vi "batch processor.vi"() -> ()   [LabVIEW 2012]
uses:
  <vilib>/Utility/miscctls.llb/LVPointTypeDef.ctl
  Private/File_location.ctl
  Public API/Post_Dust_Event.ctl
  Private/Estimate_source.ctl
  <vilib>/Utility/error.llb/DialogType.ctl
  Public API/Signal.ctl
  Private/Role ID.ctl
  Private/Hardware ID.ctl
panel:
  in  "stop 2":bool
  in  "Tab Control":enum32{"Controls", "Processing"}(tab)
  in  "Update old Errored entries?":bool
  in  "Clear IDL Errors 2":bool
  in  "Clear IDL Errors":bool
  out "Warning:":string
  out "Move Errors":errorcluster
  out "IDL Errors":errorcluster
  out "Test":bool caption="Test Database in use:"
  out "Test 2":bool=TRUE caption="Production Database in use:"
  out "Events being processed:":i32
  out "Processing Frequency (Hz):":dbl
  out "Database Update Progress:":u8(slide) scale=0.0..100.0
  out "IDL Code Executing":bool=TRUE
  out "Estimated IDL Progress:":u8(slide) scale=0.0..100.0
  in  "Update old database entries?":bool
  in  "Upper Timestamp\nFor Old Data":timestamp
  in  "Lower Timestamp\nFor Old Data":timestamp
  out "Running Old Data:":bool
  out "standard error":string
  out "standard output":string
  out "Passed":i32
  out "Quality":ext format="%.2f"
  out "Charge":ext
  out "Velocity":ext
  out "Source":i32
  out "Time taken by IDL per shot: (s)":dbl
  out "Shot being processed:":string
  out "Remaining Shots:":string
  out "Output to IDL command line:":string
  in  "stop":bool
  out "Radius":dbl
  out "Mass":ext
  out "Dust Event ID":i64
  out "High Voltage":sgl
  # "CCLDAS Database Update System V1.0"
  # "Error Status:"
  # "Beamline length change: 1:00:00.000 PM\n                                                       3/5/2014"
  # "ODBC Connection Status:"
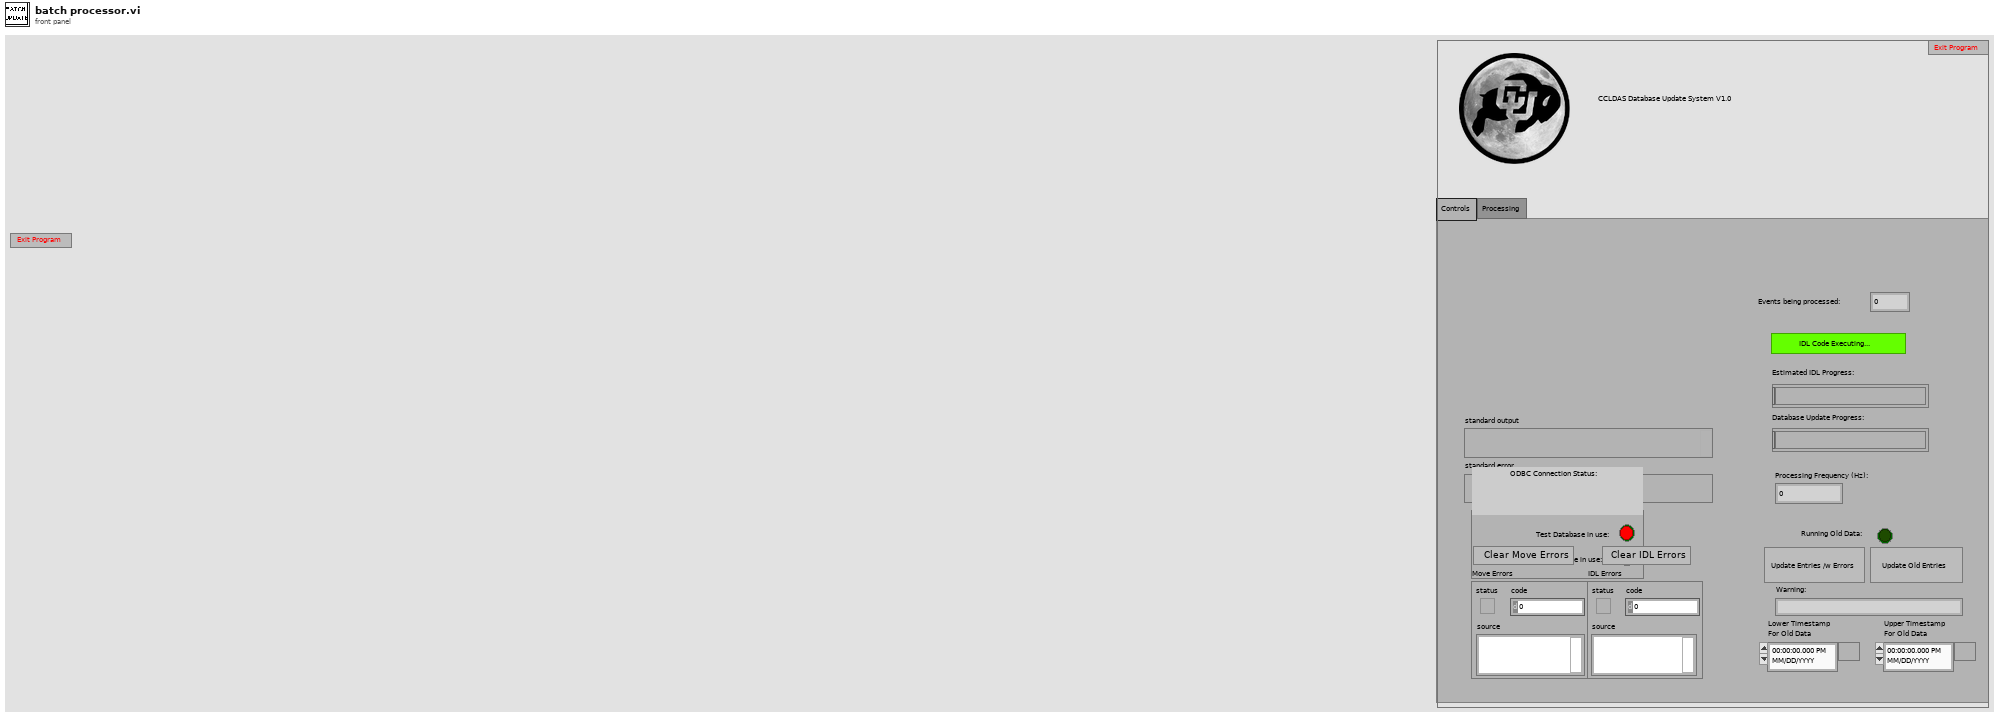
[diagram p1: front panel]
types:
  T1 = typedef "LVPointTypeDef.ctl" = cluster{"Horizontal":i16, "Vertical":i16}
  T2 = enum16{"open", "replace", "create", "open or create", "replace or create", "replace or create with confirmation"}
  T3 = typedef "Post_Dust_Event.ctl" = cluster{"Dust Event ID":i64, "Integer Timestamp":i64, "Velocity":sgl, "Mass":sgl, "Charge":sgl, "Radius":sgl, "Passed_3rd_Detector":i8, "Experiment Settings":dbl, "Pelletron ID":i32, "Estimate Source":T4, "Estimate Quality":sgl, "File Location":T5, "id_dust_info":dbl}
  T4 = typedef "Estimate_source.ctl" = i8
  T5 = typedef "File_location.ctl" = i8
  T6 = typedef "bp_cluster.ctl" = cluster{"Dust Event ID":i64, "High Voltage":sgl, "Experiment Settings  ID":i64, "File Location":T5, "Dust Density":dbl}
  T7 = enum8{"Enabled", "Disabled", "Disabled and Grayed Out"}
  T8 = typedef "Signal.ctl" = cluster{"Signal ID":i64, "Time Stamp":timestamp, "Dust Event ID":i64, "Role ID":T9, "Data":sgl[], "Signal Length":i32, "dt":sgl, "Offset":dbl, "Hardware ID":T10}
  T9 = typedef "Role ID.ctl" = enum16{"First_Detector", "Second_Detector", "Third_Detector", "LeCroy_CH1", "LeCroy_CH2", "LeCroy_CH3", "LeCroy_CH4", "PSU"}
  T10 = typedef "Hardware ID.ctl" = enum16{"Unknown", "CSA 1", "CSA 2", "CSA 3", "CSA 4", "CSA 5", "CSA 6"}
  T11 = typedef "DialogType.ctl" = u16
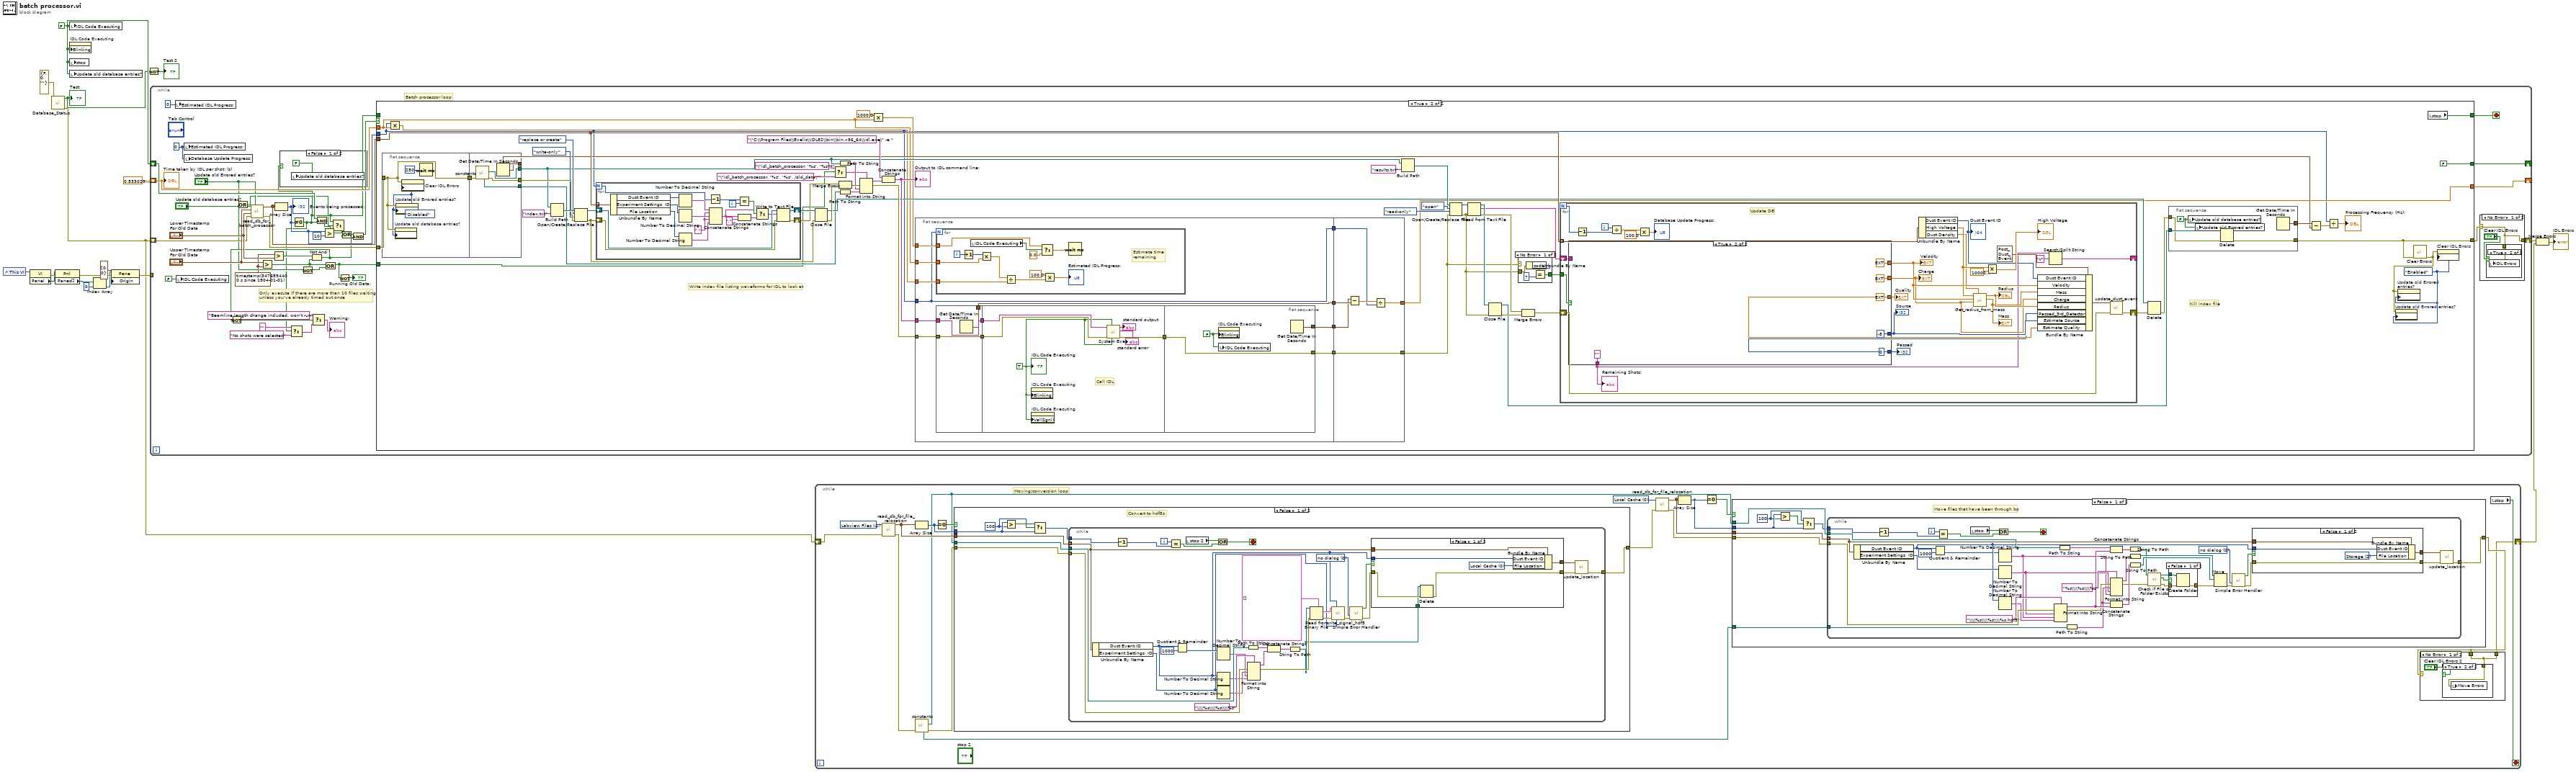
[diagram p0: block diagram]
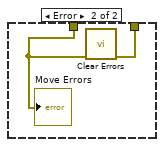
[diagram p3: hidden frame]
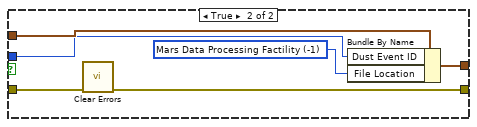
[diagram p4: hidden frame]
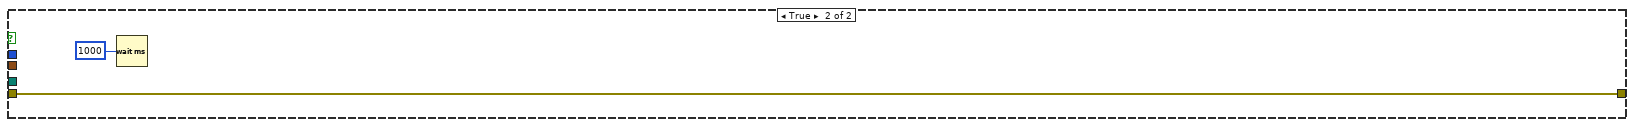
[diagram p5: hidden frame]
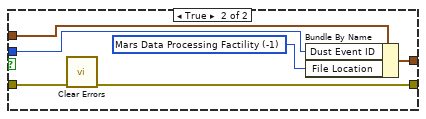
[diagram p6: hidden frame]
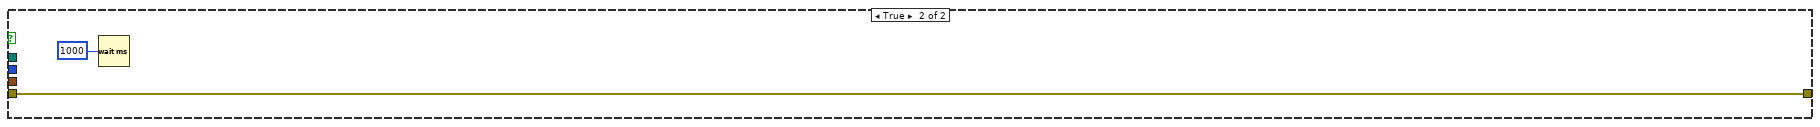
[diagram p8: hidden frame]
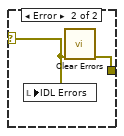
[diagram p10: hidden frame]
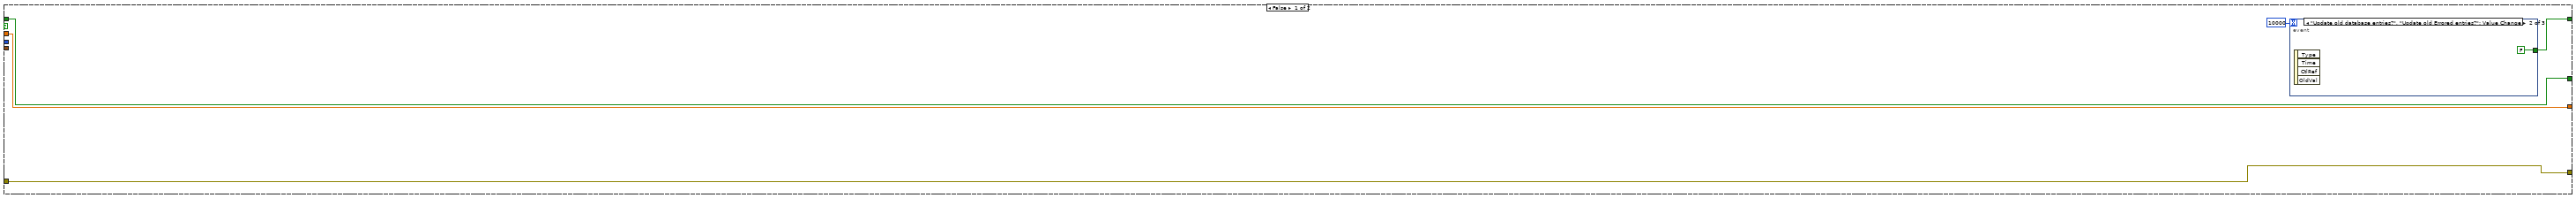
[diagram p12: hidden frame]
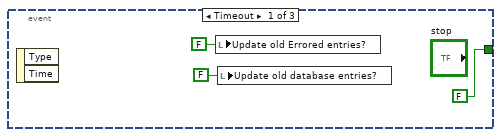
[diagram p13: hidden frame]
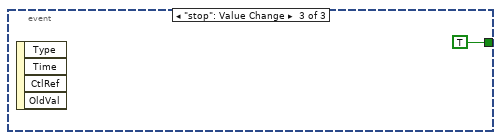
[diagram p14: hidden frame]
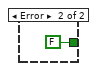
[diagram p15: hidden frame]
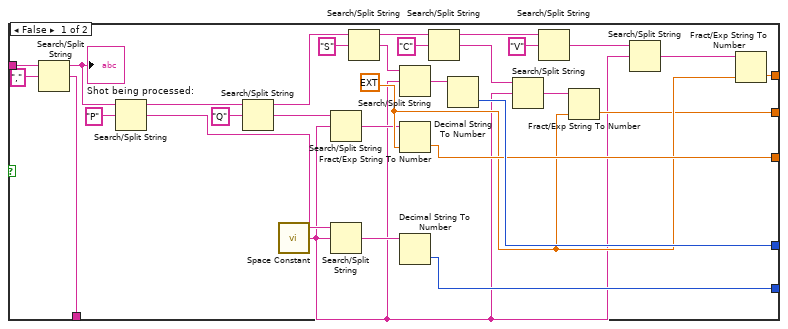
[diagram p16: hidden frame]
diagram:
  w18 = FALSE ("IDL Code Executing")
  n1 = control-ref of="This VI"() -> (w13:refnum<vi>)
  n2 = property class="VI"(reference=w13) -> (error out=w12:errorcluster, "Panel"=w11:refnum<vi>)  [unwired: 1 in, 1 out]
  n3 = call "Database_Status.vi"("error in (no error)"=errorcluster {"status"=FALSE, "code"=0, "source"=""}) -> ("error out"=w3:errorcluster, "Test Database"=w15:bool)  [unwired: 9 in]
  "Test" <- w15
  n4 = property class="Pnl"(reference=w11, error in=w12) -> (error out=w10:errorcluster, "Panes[]"=w9:refnum<vi>[])  [unwired: 1 out]
  n5 = local write "IDL Code Executing"(w18) -> ()
  n6 = property on="IDL Code Executing" class="Bool (strict)"("Blinking"=w18) -> ()  [unwired: 2 in, 2 out]
  n7 = local write "stop"(w18) -> ()
  n8 = local write "Update old database entries?"(w18) -> ()
  n9 = Index Array(array=w9, index=0) -> (element=w7:refnum<vi>)
  n10 = property class="Pane"(reference=w7, error in=w10, "Origin"=T1 {"Horizontal"=0, "Vertical"=0}) -> (error out=w5:errorcluster)  [unwired: 1 out]
  n11 = Not(x=w15) -> (.not. x?=→"Test 2":bool)
  n12 = while {
    shift-right: [w52] -> _
    shift-left: sgl 0.53303 ("y") -> [w53]
    shift-right: [w47] -> _
    shift-left: w18 -> [w48]
    tunnel: w5 -> [_]
    shift-right: [w19] -> w2
    shift-left: w3 -> [w28]
    stop <- w50 stop-if-true
    w42 = timestamp(3476894400 s since 1904-01-01) ("y")
    w54 = u8 0 ("Database Update Progress")
    # "Only execute if there are more than 10 files waiting \nunless you've already timed out once"
    # "Batch processor loop"
    n13 = local write "Estimated IDL Progress:"(u8 0 ("Estimated IDL Progress")) -> ()
    n14 = local write "IDL Code Executing"(FALSE ("IDL Code Executing")) -> ()
    n15 = local write "Estimated IDL Progress:"(w54) -> ()
    n16 = local write "Database Update Progress:"(w54) -> ()
    n17 = Or(x="Update old Errored entries?", y="Update old database entries?") -> (x .or. y?=w21:bool)
    n18 = call "read_db_for_batch_processor.vi"("Update Error files?"="Update old Errored entries?", "error in (no error)"=w28, "Lower Timestamp"="Lower Timestamp\nFor Old Data", "Upper Timestamp"="Upper Timestamp\nFor Old Data", "Update old files?"=w21) -> ("error out"=w57:errorcluster, "BP Array"=w56:T6[])  [unwired: 5 in]
    n19 = Greater?(x="Upper Timestamp\nFor Old Data", y=w42) -> (0:w38:bool)
    n20 = Greater?(x=w42, y="Lower Timestamp\nFor Old Data") -> (0:w39:bool)
    n21 = Array Size(array=w56) -> (size(s)=w45:i32)
    "Events being processed:" <- w45
    n22 = Not Equal To 0?(x=w45) -> (x != 0?=w24:bool)
    n23 = case shown="False" w24 {
      frame False {
        n24 = local write "Update old database entries?"(FALSE ("Update old database entries?")) -> ()
      }
      frame True {
      }
    }
    n25 = Select(t="" ("Warning:"), s=w24, f="No shots were selected") -> (s? t:f=w33:string)
    n26 = Not(x="Update old database entries?") -> (.not. x?=w29:bool)
    n27 = Not And(1:w38, 2:w39) -> (0:w37:bool)
    n28 = Not(x=w37) -> (.not. x?=w34:bool)
    n29 = Select(t="Beamline length change included, won't run" ("Warning:"), s=w34, f=w33) -> (s? t:f=→"Warning:":string)
    n30 = And(x=w48, y=w24) -> (x .and. y?=w25:bool)
    n31 = Greater?(x=w45, y=10) -> (0:w46:bool)
    n32 = Or(x=w38, y=w29) -> (x .or. y?=w30:bool)
    n33 = Select(t=w24, s=w21, f=w25) -> (s? t:f=w26:bool)
    n34 = Not(x=w30) -> (.not. x?=→"Running Old Data:":bool)
    n35 = Or(x=w46, y=w26) -> (x .or. y?=w44:bool)
    n36 = And(x=w44, y=w37) -> (x .and. y?=w40:bool)
    n37 = case shown="True" w40 {
      tunnel: w57 -> [w64 w133]
      tunnel: [w64 w79] -> w20
      tunnel: w56 -> [_ w135]
      tunnel: w45 -> [_ w84]
      tunnel: w53 -> [w68 w96]
      tunnel: [w68 w92] -> w52
      tunnel: [w66 w89] -> w50
      tunnel: [w65 FALSE ("Update all files?")] -> w47
      tunnel: w24 -> [w65 _]
      tunnel: w30 -> [_ w80]
      frame False {
        n38 = event shown="[1] \"Update old database entries?\", \"Update old Errored entries?\": Value Change" {
          selector: _ -> [_ _ _]
          dyn-events: _ -> [_ _ _]
          timeout: u32 10000 ("milliseconds to wait") -> [_ _ _]
          tunnel: [FALSE FALSE TRUE] -> w66
          event Timeout {
            n39 = event-data() -> ()  [unwired: 1 in, 2 out]
            n40 = local write "Update old Errored entries?"(FALSE ("Update old Errored entries?")) -> ()
            n41 = local write "Update old database entries?"(FALSE ("Update old database entries?")) -> ()
          }
          event "Update old database entries?", "Update old Errored entries?": Value Change {
            n42 = event-data() -> ()  [unwired: 1 in, 4 out]
          }
          event "stop": Value Change {
            n43 = event-data() -> ()  [unwired: 1 in, 4 out]
          }
        }
      }
      frame True {
        w74 = T7."Enabled" ("Disabled")
        # "Kill index file"
        # "Write index file listing waveforms for IDL to look at"
        n44 = flat-sequence {
          tunnel: w133 -> [w142]
          tunnel: [w142] -> w88
          tunnel: [w147] -> w129
          tunnel: [w146] -> w108
          tunnel: [w145] -> w100
          tunnel: w88 -> [w148]
          tunnel: [w144] -> w86
          frame #0 {
            w141 = T7."Disabled" ("Disabled")
            n45 = property on="Update old database entries?" class="Bool (strict)"(error in=w142, "DisabledEnum"=w141) -> ()  [unwired: 1 in, 2 out]
            n46 = property on="Update old Errored entries?" class="Bool (strict)"(error in=w142, "DisabledEnum"=w141) -> ()  [unwired: 1 in, 2 out]
            n47 = property on="Clear IDL Errors" class="Bool"(error in=w142, "DisabledEnum"=w141) -> ()  [unwired: 1 in, 2 out]
            n48 = Wait (ms)(milliseconds to wait=u32 250) -> ()  [unwired: 1 out]
          }
          frame #1 {
            n49 = call "constants.vi"("error in (no error)"=w148) -> ("error out"=w147:errorcluster, "file path for Signal .hdf5 files"=w146:path, "file path for Processed Signal .hdf5 files"=w144:path)  [unwired: 4 in, 4 out]
            n50 = Get Date/Time In Seconds() -> (seconds since 1Jan1904=w145:timestamp)
          }
        }
        n51 = Multiply(x=w84, y=w96) -> (x*y=w98:dbl)
        n52 = Build Path(base path=w108, name or relative path="index.txt") -> (appended path=w132:path)
        n53 = Open/Create/Replace File(file path (use dialog)=w132, error in=w129, operation (0:open)=T2."replace or create", access (0:read/write)=enum16{"read/write", "read-only", "write-only"}."write-only") -> (refnum out=w131:refnum<file>, error out=w128:errorcluster)  [unwired: 2 in, 1 out]
        n54 = for {
          N: w84 -> [w207]
          shift-right: [w214] -> w127
          shift-left: w128 -> [w213]
          tunnel: w135 -> [w215] mode=indexing
          shift-right: [w211] -> w130
          shift-left: w131 -> [w212]
          i -> [w210]
          w197 = " " ("string")
          n55 = Unbundle By Name(w215) -> ("Dust Event ID"=w199:i64, "Experiment Settings  ID"=w205:i64, "File Location"=w198:T5)
          n56 = Number To Decimal String(number=w199) -> (decimal integer string=w201:string)  [unwired: 1 in]
          n57 = Number To Decimal String(number=w205) -> (decimal integer string=w204:string)  [unwired: 1 in]
          n58 = Number To Decimal String(number=w198) -> (decimal integer string=w196:string)  [unwired: 1 in]
          n59 = Decrement(x=w207) -> (x-1=w206:i32)
          n60 = Concatenate Strings(w201, w197, w204, w197, w196) -> (w200:string)
          n61 = Equal?(x=w206, y=w210) -> (x = y?=w209:bool)
          n62 = Concatenate Strings(w200, "," ("string")) -> (w202:string)
          n63 = Select(t=w200, s=w209, f=w202) -> (s? t:f=w208:string)
          n64 = Write to Text File(file (use dialog)=w212, text=w208, error in=w213) -> (refnum out=w211:refnum<file>, error out=w214:errorcluster)  [unwired: 1 in, 1 out]
        }
        n65 = Close File(refnum=w130, error in=w128) -> (path=w106:path, error out=w126:errorcluster)
        n66 = Select(t="\"idl_batch_processor, '%s', '%s'\"" ("format string"), s=w80, f="\"idl_batch_processor, '%s', '%s', /old_data\"" ("format string")) -> (s? t:f=w82:string)
        n67 = Path To String(path=w108) -> (string=w109:string)
        n68 = Path To String(path=w86) -> (string=w85:string)
        n69 = Merge Errors(w127, w126) -> (w115:errorcluster)
        n70 = Format Into String(format string=w82, error in=w115, w109, w85) -> (resulting string=w124:string, error out=w116:errorcluster)  [unwired: 1 in]
        n71 = Multiply(x=sgl 1000.0 ("y"), y=w96) -> (x*y=w97:dbl)
        n72 = Concatenate Strings("\"C:\\Program Files\\Exelis\\IDL82\\bin\\bin.x86_64\\idl.exe\" -e ", w124) -> (w123:string)
        "Output to IDL command line:" <- w123
        n73 = flat-sequence {
          tunnel: [w154] -> w94
          tunnel: [w160] -> w93
          tunnel: [w159] -> w91
          tunnel: [w158] -> w90
          tunnel: w84 -> [w160]
          tunnel: w97 -> [w161]
          tunnel: w96 -> [w162]
          tunnel: w98 -> [w163]
          tunnel: w116 -> [w164]
          tunnel: w123 -> [w165]
          tunnel: w94 -> [w195]
          tunnel: w93 -> [w193]
          tunnel: [w192] -> w92
          tunnel: w91 -> [w191]
          tunnel: [w191] -> w78
          tunnel: w90 -> [w190]
          frame #0 {
            n74 = for {
              N: w160 -> [_]
              tunnel: w163 -> [w173]
              tunnel: w162 -> [w176]
              tunnel: w161 -> [w167]
              i -> [w177]
              # "Estimate time \nremaining"
              n75 = Increment(x=w177) -> (x+1=w175:i32)
              n76 = local read "IDL Code Executing"() -> (w169:bool)
              n77 = Multiply(x=w175, y=w176) -> (x*y=w174:dbl)
              n78 = Divide(x=w174, y=w173) -> (x/y=w172:dbl)
              n79 = Select(t=w167, s=w169, f=0.0) -> (s? t:f=w168:dbl)
              n80 = Multiply(x=sgl 100.0, y=w172) -> (x*y=→"Estimated IDL Progress:":dbl)
              n81 = Wait (ms)(milliseconds to wait=w168) -> ()  [unwired: 1 out]
            }
            n82 = flat-sequence {
              tunnel: w164 -> [w179]
              tunnel: w165 -> [w180]
              tunnel: [w180] -> w156
              tunnel: [w179] -> w155
              tunnel: [w178] -> w154
              tunnel: [w184] -> w157
              tunnel: w156 -> [w186]
              tunnel: w155 -> [w185]
              tunnel: [w188] -> w158
              tunnel: [w189] -> w159
              tunnel: w157 -> [w189]
              frame #0 {
                n83 = Get Date/Time In Seconds() -> (seconds since 1Jan1904=w178:timestamp)
              }
              frame #1 {
                w183 = TRUE ("wait until completion? (T)")
                # "Call IDL"
                n84 = property on="IDL Code Executing" class="Bool (strict)"("Blinking"=w183) -> ()  [unwired: 2 in, 2 out]
                n85 = property on="IDL Code Executing" class="Bool (strict)"("Val(Sgnl)"=w183) -> ()  [unwired: 2 in, 2 out]
                n86 = call <vilib>:"System Exec.vi"("run minimized? (F)"=w183, "wait until completion? (T)"=w183, "error in (no error)"=w185, "command line"=w186) -> ("error out"=w184:errorcluster, "standard error"=→"standard error":string, "standard output"=→"standard output":string)  [unwired: 4 in, 1 out]
                "IDL Code Executing" <- w183
              }
              frame #2 {
                w187 = FALSE ("IDL Code Executing")
                n87 = property on="IDL Code Executing" class="Bool (strict)"("Blinking"=w187) -> ()  [unwired: 2 in, 2 out]
                n88 = local write "IDL Code Executing"(w187) -> ()
                n89 = Get Date/Time In Seconds() -> (seconds since 1Jan1904=w188:timestamp)
              }
            }
          }
          frame #1 {
            n90 = Subtract(x=w190, y=w195) -> (x-y=w194:dbl)
            n91 = Divide(x=w194, y=w193) -> (x/y=w192:dbl)
          }
        }
        n92 = Build Path(base path=w108, name or relative path="results.txt") -> (appended path=w121:path)
        n93 = Open/Create/Replace File(file path (use dialog)=w121, error in=w78, operation (0:open)=T2."open", access (0:read/write)=enum16{"read/write", "read-only", "write-only"}."read-only") -> (refnum out=w120:refnum<file>, error out=w77:errorcluster)  [unwired: 2 in, 1 out]
        n94 = Read from Text File(file (use dialog)=w120, error in=w77) -> (refnum out=w110:refnum<file>, text=w107:string, error out=w119:errorcluster)  [unwired: 2 in, 1 out]
        n95 = Close File(refnum=w110, error in=w77) -> (path=w105:path, error out=w118:errorcluster)
        n96 = case shown="No Error" w78 {
          tunnel: w77 -> [w139 _]
          tunnel: [w136 FALSE] -> w76
          frame No Error {
            n97 = Unbundle By Name(w139) -> ("code"=w138:i32)
            n98 = Equal?(x=w138, y=7) -> (x = y?=w136:bool)
          }
          frame Error {
          }
        }
        n99 = Merge Errors(w119, w118) -> (w117:errorcluster)
        n100 = for {
          N -> [w223]
          shift-right: [w235] -> w103
          shift-left: w117 -> [w228]
          tunnel: w135 -> [w243] mode=indexing
          shift-right: [w220] -> _
          shift-left: w107 -> [w229]
          tunnel: w76 -> [w216]
          i -> [w227]
          # "Update DB"
          n101 = case shown="True" w216 {
            tunnel: [w261 -5] -> w242
            tunnel: [w260 ext 0.0] -> w241
            tunnel: [w258 0] -> w240
            tunnel: [w257 ext -5.0] -> w232
            tunnel: [w256 ext -5.0] -> w231
            tunnel: w229 -> [w255 _]
            tunnel: [w249 ""] -> w221
            frame False {
              w259 = ext 0.0 ("default (0 I32)")
              n102 = Search/Split String(string=w255, search string/char (-)=",") -> (substring before match=w254:string, match + rest of string=w249:string)  [unwired: 1 in, 1 out]
              "Shot being processed:" <- w254
              n103 = Search/Split String(string=w254, search string/char (-)="P") -> (substring before match=w271:string, match + rest of string=w272:string)  [unwired: 1 in, 1 out]
              n104 = Search/Split String(string=w271, search string/char (-)="Q") -> (substring before match=w268:string, match + rest of string=w269:string)  [unwired: 1 in, 1 out]
              n105 = call <vilib>:"Space Constant.vi"() -> ("String"=w245:string)
              n106 = Search/Split String(string=w269, search string/char (-)=w245) -> (match + rest of string=w246:string)  [unwired: 1 in, 2 out]
              n107 = Search/Split String(string=w272, search string/char (-)=w245) -> (match + rest of string=w248:string)  [unwired: 1 in, 2 out]
              n108 = Search/Split String(string=w268, search string/char (-)="S") -> (substring before match=w244:string, match + rest of string=w266:string)  [unwired: 1 in, 1 out]
              n109 = Search/Split String(string=w266, search string/char (-)=w245) -> (match + rest of string=w247:string)  [unwired: 1 in, 2 out]
              n110 = Fract/Exp String To Number(string=w246, default (0 dbl)=w259) -> (number=w260:ext)  [unwired: 2 in, 1 out]
              n111 = Decimal String To Number(string=w248) -> (number=w258:i32)  [unwired: 2 in, 1 out]
              n112 = Search/Split String(string=w244, search string/char (-)="C") -> (substring before match=w265:string, match + rest of string=w262:string)  [unwired: 1 in, 1 out]
              n113 = Decimal String To Number(string=w247) -> (number=w261:i32)  [unwired: 2 in, 1 out]
              n114 = Search/Split String(string=w262, search string/char (-)=w245) -> (match + rest of string=w252:string)  [unwired: 1 in, 2 out]
              n115 = Search/Split String(string=w265, search string/char (-)="V") -> (match + rest of string=w263:string)  [unwired: 1 in, 2 out]
              n116 = Fract/Exp String To Number(string=w252, default (0 dbl)=w259) -> (number=w256:ext)  [unwired: 2 in, 1 out]
              n117 = Search/Split String(string=w263, search string/char (-)=w245) -> (match + rest of string=w251:string)  [unwired: 1 in, 2 out]
              n118 = Fract/Exp String To Number(string=w251, default (0 dbl)=w259) -> (number=w257:ext)  [unwired: 2 in, 1 out]
            }
            frame True {
            }
          }
          "Passed" <- w240
          "Quality" <- w241
          "Charge" <- w231
          "Velocity" <- w232
          "Remaining Shots:" <- w221
          "Source" <- w242
          n119 = Decrement(x=w223) -> (x-1=w222:i32)
          n120 = Divide(x=w227, y=w222) -> (x/y=w226:dbl)
          n121 = Multiply(x=w226, y=100.0) -> (x*y=→"Database Update Progress:":dbl)
          n122 = Unbundle By Name(w243) -> ("Dust Event ID"=w234:i64, "High Voltage"=w233:sgl, "Dust Density"=w217:dbl)
          "Dust Event ID" <- w234
          n123 = call "Get_radius_from_mass.vi"("Density"=w217, "Charge"=w231, "Velocity"=w232, "High Voltage (MV)"=w233) -> ("Mass"=w230:ext, "Radius"=w239:dbl)  [unwired: 6 in]
          "Mass" <- w230
          "Radius" <- w239
          n124 = Multiply(x=w233, y=sgl 1000000.0) -> (x*y=→"High Voltage":sgl)
          n125 = Bundle By Name(cluster=T3 {"Dust Event ID"=0, "Integer Timestamp"=0, "Velocity"=0.0, "Mass"=0.0, "Charge"=0.0, "Radius"=0.0, "Passed_3rd_Detector"=0, "Experiment Settings"=0.0, "Pelletron ID"=0, "Estimate Source"=0, "Estimate Quality"=0.0, "File Location"=0, "id_dust_info"=0.0} ("Cluster"), "Dust Event ID"=w234, "Velocity"=w232, "Mass"=w230, "Charge"=w231, "Radius"=w239, "Passed_3rd_Detector"=w240, "Estimate Source"=w242, "Estimate Quality"=w241) -> (w218:T3)
          n126 = Search/Split String(string=w221, search string/char (-)="V") -> (match + rest of string=w220:string)  [unwired: 1 in, 2 out]
          n127 = call "update_dust_event.vi"("error in (no error)"=w228, "Cluster"=w218) -> ("error out"=w235:errorcluster)  [unwired: 8 in, 1 out]
        }
        n128 = Delete(path (use dialog)=w106, error in=w103) -> (error out=w104:errorcluster)  [unwired: 3 in, 2 out]
        n129 = flat-sequence {
          tunnel: w105 -> [w153]
          tunnel: w104 -> [w152]
          tunnel: [w151] -> w79
          tunnel: [w150] -> w101
          frame #0 {
            w149 = FALSE ("Update all files?")
            n130 = local write "Update old database entries?"(w149) -> ()
            n131 = local write "Update old Errored entries?"(w149) -> ()
            n132 = Delete(path (use dialog)=w153, error in=w152) -> (error out=w151:errorcluster)  [unwired: 3 in, 2 out]
            n133 = Get Date/Time In Seconds() -> (seconds since 1Jan1904=w150:timestamp)
          }
        }
        n134 = Subtract(x=w101, y=w100) -> (x-y=w102:dbl)
        n135 = Divide(x=w84, y=w102) -> (x/y=→"Processing Frequency (Hz):":dbl)
        n136 = call <vilib>:"Clear Errors.vi"("error in (no error)"=w79) -> ("error out"=w75:errorcluster)  [unwired: 6 in]
        n137 = property on="Update old Errored entries?" class="Bool (strict)"(error in=w75, "DisabledEnum"=w74) -> ()  [unwired: 1 in, 2 out]
        n138 = property on="Update old Errored entries?" class="Bool (strict)"(error in=w75, "DisabledEnum"=w74) -> ()  [unwired: 1 in, 2 out]
        n139 = local read "stop"() -> (w89:bool)
        n140 = property on="Clear IDL Errors" class="Bool"(error in=w75, "DisabledEnum"=w74) -> ()  [unwired: 1 in, 2 out]
      }
    }
    n141 = case shown="No Error" w20 {
      selector: w20 -> [w58 w62]
      tunnel: [w58 w61] -> w19
      frame No Error {
        n142 = case shown="True" "Clear IDL Errors" {
          tunnel: w58 -> [_ w60]
          frame False {
          }
          frame True {
            n143 = local write "IDL Errors"(w60) -> ()
          }
        }
      }
      frame Error {
        n144 = local write "IDL Errors"(w62) -> ()
        n145 = call <vilib>:"Clear Errors.vi"("error in (no error)"=w62) -> ("error out"=w61:errorcluster)  [unwired: 6 in]
      }
    }
    "Time taken by IDL per shot: (s)" <- w53
  }
  n146 = while {
    shift-right: [w280] -> w4
    shift-left: w3 -> [w282]
    stop <- w297 stop-if-true
    w287 = T5 -2 items=["Labview Files"=-2, "Mars Data Processing Factility"=-1, "Local Cache "=0, "Old Storage"=1, "Storage"=2] ("File Location")
    w293 = T5 0 items=["Labview Files"=-2, "Mars Data Processing Factility"=-1, "Local Cache "=0, "Old Storage"=1, "Storage"=2] ("File Location")
    # "Moving/conversion loop"
    n147 = call "read_db_for_file_relocation.vi"("error in (no error)"=w282, "File Location"=w287) -> ("error out"=w292:errorcluster, "BP Array"=w290:T6[])  [unwired: 8 in]
    n148 = Array Size(array=w290) -> (size(s)=w288:i32)
    n149 = call "constants.vi"("error in (no error)"=w292) -> ("error out"=w291:errorcluster, "file path for Signal .hdf5 files"=w285:path, "file path for Processed Signal .hdf5 files"=w284:path)  [unwired: 4 in, 4 out]
    n150 = Equal To 0?(x=w288) -> (x = 0?=w289:bool)
    n151 = case shown="False" w289 {
      tunnel: w291 -> [w310 w356]
      tunnel: w285 -> [w309 _]
      tunnel: w290 -> [w308 _]
      tunnel: w288 -> [w304 _]
      tunnel: [w307 w356] -> w286
      frame False {
        w303 = 100 ("y")
        # "Convert to hdf5s"
        n152 = Greater?(x=w304, y=w303) -> (0:w306:bool)
        n153 = Select(t=w303, s=w306, f=w304) -> (s? t:f=w305:i32)
        n154 = while {
          tunnel: w308 -> [w341] mode=indexing
          tunnel: w309 -> [w339]
          tunnel: w305 -> [w330]
          tunnel: w310 -> [w328]
          tunnel: [w342] -> w307
          i -> [w331]
          stop <- w334 stop-if-true
          w325 = T11 0 items=["no dialog", "OK message", "continue or stop message", "OK message + warnings", "continue/stop + warnings"] ("type of dialog (OK msg:1)")
          n155 = Unbundle By Name(w341) -> ("Dust Event ID"=w313:i64, "Experiment Settings  ID"=w312:i64)
          n156 = Decrement(x=w330) -> (x-1=w332:i32)
          n157 = Equal?(x=w331, y=w332) -> (x = y?=w329:bool)
          n158 = Quotient & Remainder(x=w313, y=i64 1000) -> (floor(x/y)=w321:i64)  [unwired: 1 out]
          n159 = local read "stop 2"() -> (w333:bool)
          n160 = Or(x=w333, y=w329) -> (x .or. y?=w334:bool)
          n161 = Number To Decimal String(number=w321) -> (decimal integer string=w319:string)  [unwired: 1 in]
          n162 = Number To Decimal String(number=w313) -> (decimal integer string=w322:string)  [unwired: 1 in]
          n163 = Number To Decimal String(number=w312) -> (decimal integer string=w327:string)  [unwired: 1 in]
          n164 = Path To String(path=w339) -> (string=w335:string)
          n165 = Format Into String(format string="\\\\%s\\\\%s\\\\%s", error in=w328, w327, w319, w322) -> (resulting string=w336:string, error out=w318:errorcluster)  [unwired: 1 in]
          n166 = Concatenate Strings(w335, w336) -> (w338:string)
          n167 = String To Path(string=w338) -> (path=w311:path)
          n168 = Read from Binary File(5:T8[] [] ("Signal array"), 8:w318, 11:w311) -> (0:w317:errorcluster, 2:w314:T8[])  [unwired: 3 in, 2 out]
          n169 = call "write_signal_hdf5.vi"("Experiment Settings ID"=w312, "Index"=w313, "error in"=w317, "Signal array"=w314) -> ("error out"=w316:errorcluster)  [unwired: 6 in, 1 out]
          n170 = call <vilib>:"Simple Error Handler.vi"("type of dialog (OK msg:1)"=w325, "error in (no error)"=w316) -> ("error?"=w326:bool, "error out"=w324:errorcluster)  [unwired: 3 in, 3 out]
          n171 = case shown="False" w326 {
            tunnel: w341 -> [w349 w355]
            tunnel: [w348 w352] -> w340
            tunnel: w313 -> [w347 w354]
            tunnel: [w345 w351] -> w323
            tunnel: w324 -> [w344 w350]
            tunnel: w311 -> [w343 _]
            frame False {
              w346 = T5 0 items=["Labview Files"=-2, "Mars Data Processing Factility"=-1, "Local Cache "=0, "Old Storage"=1, "Storage"=2] ("File Location")
              n172 = Delete(path (use dialog)=w343, error in=w344) -> (error out=w345:errorcluster)  [unwired: 3 in, 2 out]
              n173 = Bundle By Name(cluster=w349, "Dust Event ID"=w347, "File Location"=w346) -> (w348:T6)
            }
            frame True {
              w353 = T5 -1 items=["Mars Data Processing Factility"=-1, "Local Cache "=0, "Storage"=1] ("File Location")
              n174 = call <vilib>:"Clear Errors.vi"("error in (no error)"=w350) -> ("error out"=w351:errorcluster)  [unwired: 6 in]
              n175 = Bundle By Name(cluster=w355, "Dust Event ID"=w354, "File Location"=w353) -> (w352:T6)
            }
          }
          n176 = call "update_location.vi"("error in (no error)"=w323, "Batch Processing Cluster"=w340) -> ("error out"=w342:errorcluster)  [unwired: 8 in, 1 out]
        }
      }
      frame True {
        n177 = Wait (ms)(milliseconds to wait=u32 1000) -> ()  [unwired: 1 out]
      }
    }
    n178 = call "read_db_for_file_relocation.vi"("error in (no error)"=w286, "File Location"=w293) -> ("error out"=w283:errorcluster, "BP Array"=w296:T6[])  [unwired: 8 in]
    n179 = Array Size(array=w296) -> (size(s)=w294:i32)
    n180 = Equal To 0?(x=w294) -> (x = 0?=w295:bool)
    n181 = case shown="False" w295 {
      tunnel: w283 -> [w366 w423]
      tunnel: w284 -> [w365 _]
      tunnel: w285 -> [w364 _]
      tunnel: w296 -> [w363 _]
      tunnel: w294 -> [w359 _]
      tunnel: [w362 w423] -> w281
      frame False {
        w358 = 100 ("y")
        # "Move files that have been through bp"
        n182 = Greater?(x=w359, y=w358) -> (0:w361:bool)
        n183 = Select(t=w358, s=w361, f=w359) -> (s? t:f=w360:i32)
        n184 = while {
          tunnel: w363 -> [w406] mode=indexing
          tunnel: w365 -> [w402]
          tunnel: w364 -> [w403]
          tunnel: w360 -> [w391]
          tunnel: w366 -> [w389]
          tunnel: [w407] -> w362
          i -> [w392]
          stop <- w395 stop-if-true
          w374 = T11 0 items=["no dialog", "OK message", "continue or stop message", "OK message + warnings", "continue/stop + warnings"] ("type of dialog (OK msg:1)")
          n185 = Unbundle By Name(w406) -> ("Dust Event ID"=w370:i64, "Experiment Settings  ID"=w404:i64)
          n186 = Decrement(x=w391) -> (x-1=w393:i32)
          n187 = Quotient & Remainder(x=w370, y=i64 1000) -> (floor(x/y)=w369:i64)  [unwired: 1 out]
          n188 = Equal?(x=w392, y=w393) -> (x = y?=w390:bool)
          n189 = local read "stop"() -> (w394:bool)
          n190 = Or(x=w394, y=w390) -> (x .or. y?=w395:bool)
          n191 = Number To Decimal String(number=w369) -> (decimal integer string=w367:string)  [unwired: 1 in]
          n192 = Number To Decimal String(number=w404) -> (decimal integer string=w378:string)  [unwired: 1 in]
          n193 = Number To Decimal String(number=w370) -> (decimal integer string=w371:string)  [unwired: 1 in]
          n194 = Format Into String(format string="\\\\%s\\\\%s\\\\%s.hdf5", error in=w389, w378, w367, w371) -> (resulting string=w398:string, error out=w381:errorcluster)  [unwired: 1 in]
          n195 = Path To String(path=w403) -> (string=w397:string)
          n196 = Path To String(path=w402) -> (string=w383:string)
          n197 = Concatenate Strings(w397, w398) -> (w400:string)
          n198 = Format Into String(format string="%s\\\\%s\\\\%s", error in=w381, w383, w378, w367) -> (resulting string=w382:string, error out=w380:errorcluster)  [unwired: 1 in]
          n199 = Concatenate Strings(w383, w398) -> (w401:string)
          n200 = String To Path(string=w400) -> (path=w396:path)
          n201 = String To Path(string=w382) -> (path=w377:path)
          n202 = String To Path(string=w401) -> (path=w384:path)
          n203 = call <vilib>:"Check if File or Folder Exists.vi"("error in (no error)"=w380, "path"=w377) -> ("error out"=w386:errorcluster, "file or folder exists?"=w388:bool, "dup path"=w387:path)  [unwired: 7 in]
          n204 = case shown="False" w388 {
            tunnel: w387 -> [w421 _]
            tunnel: w386 -> [w420 w422]
            tunnel: [w419 w422] -> w385
            frame False {
              n205 = Create Folder(path (use dialog)=w421, error in=w420) -> (error out=w419:errorcluster)  [unwired: 1 in, 2 out]
            }
            frame True {
            }
          }
          n206 = Move(source path=w396, error in=w385, 10:w384) -> (error out=w376:errorcluster)  [unwired: 2 in, 2 out]
          n207 = call <vilib>:"Simple Error Handler.vi"("type of dialog (OK msg:1)"=w374, "error in (no error)"=w376) -> ("error?"=w375:bool, "error out"=w373:errorcluster)  [unwired: 3 in, 3 out]
          n208 = case shown="False" w375 {
            tunnel: w406 -> [w412 w418]
            tunnel: [w411 w415] -> w405
            tunnel: w370 -> [w410 w417]
            tunnel: [w409 w414] -> w372
            tunnel: w373 -> [w409 w413]
            frame False {
              w408 = T5 2 items=["Mars Data Processing Factility"=-1, "Local Cache "=0, "Old Storage"=1, "Storage"=2] ("File Location")
              n209 = Bundle By Name(cluster=w412, "Dust Event ID"=w410, "File Location"=w408) -> (w411:T6)
            }
            frame True {
              w416 = T5 -1 items=["Mars Data Processing Factility"=-1, "Local Cache "=0, "Storage"=1] ("File Location")
              n210 = call <vilib>:"Clear Errors.vi"("error in (no error)"=w413) -> ("error out"=w414:errorcluster)  [unwired: 6 in]
              n211 = Bundle By Name(cluster=w418, "Dust Event ID"=w417, "File Location"=w416) -> (w415:T6)
            }
          }
          n212 = call "update_location.vi"("error in (no error)"=w372, "Batch Processing Cluster"=w405) -> ("error out"=w407:errorcluster)  [unwired: 8 in, 1 out]
        }
      }
      frame True {
        n213 = Wait (ms)(milliseconds to wait=u32 1000) -> ()  [unwired: 1 out]
      }
    }
    n214 = case shown="No Error" w281 {
      tunnel: w281 -> [w298 w302]
      tunnel: [w298 w301] -> w280
      frame No Error {
        n215 = case shown="True" "Clear IDL Errors 2" {
          tunnel: w298 -> [_ w300]
          frame False {
          }
          frame True {
            n216 = local write "Move Errors"(w300) -> ()
          }
        }
      }
      frame Error {
        n217 = call <vilib>:"Clear Errors.vi"("error in (no error)"=w302) -> ("error out"=w301:errorcluster)  [unwired: 6 in]
        "Move Errors" <- w302
      }
    }
    n218 = local read "stop"() -> (w297:bool)
  }
  n219 = Merge Errors(w2, w4) -> (→"IDL Errors":errorcluster)
